vi "Conf_AI.vi"(8 "error in (no error)":errorcluster, 10 "PIN Number":i8, 11 "Driver_AI_AO in":refnum<class "Driver_AI_AO.lvclass">) -> (0 "error out":errorcluster, 3 "Driver_AI_AO out":refnum<class "Driver_AI_AO.lvclass">)   [LabVIEW 2023, in "Driver_AI_AO.lvlib" / "Driver_AI_AO.lvclass"]
uses:
  Driver_AI_AO.lvclass
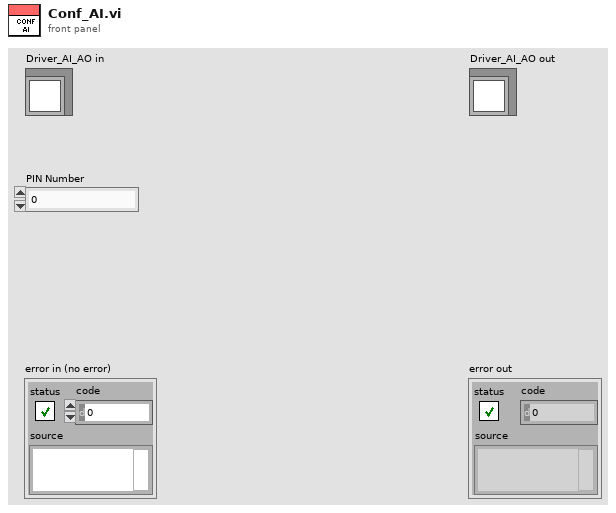
[diagram p1: front panel]
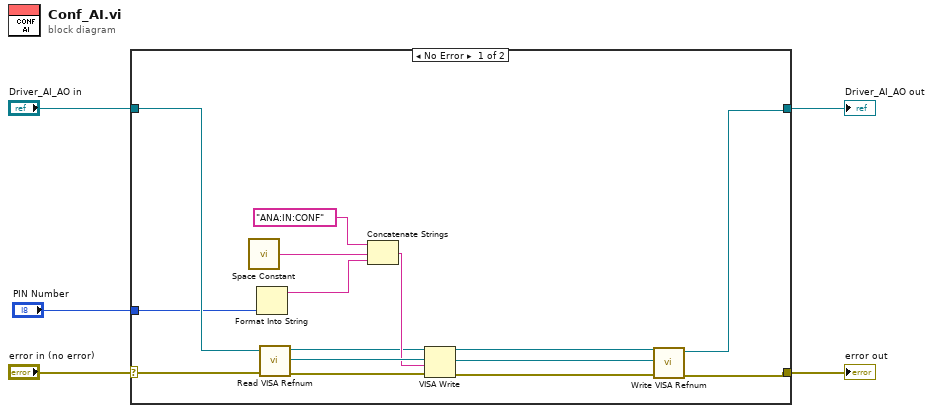
[diagram p0: block diagram]
diagram:
  n1 = case shown="No Error" "error in (no error)" {
    selector: "error in (no error)" -> [w10 w21]
    tunnel: [w9 w21] -> w4
    tunnel: [w7 w20] -> w2
    tunnel: "Driver_AI_AO in" -> [w8 w20]
    tunnel: "PIN Number" -> [w6 _]
    frame No Error {
      n2 = call <vilib>:"Space Constant.vi"() -> ("String"=w18:string)
      n3 = Format Into String(w6) -> (resulting string=w17:string)  [unwired: 3 in, 1 out]
      n4 = call-dynamic "Read VISA Refnum.vi"("error in (no error)"=w10, "Driver in"=w8) -> ("error out"=w14:errorcluster, "VISA Refnum"=w16:refnum<visa-resource-name>, "Driver out"=w12:refnum<class "Driver_AI_AO.lvclass">)  [unwired: 7 in]
      n5 = Concatenate Strings("ANA:IN:CONF", w18, w17) -> (w15:string)
      n6 = VISA Write(VISA resource name=w16, write buffer=w15, error in (no error)=w14) -> (VISA resource name out=w11:refnum<visa-resource-name>, error out=w13:errorcluster)  [unwired: 1 out]
      n7 = call-dynamic "Write VISA Refnum.vi"("error in (no error)"=w13, "VISA Refnum"=w11, "Driver in"=w12) -> ("error out"=w9:errorcluster, "Driver out"=w7:refnum<class "Driver_AI_AO.lvclass">)  [unwired: 7 in]
    }
    frame Error {
    }
  }
  "error out" <- w4
  "Driver_AI_AO out" <- w2
